vi "Run.vi"(8 "error in (no error)":errorcluster, 11 "Generic Plugin in":refnum<class "Generic Plugin.lvclass">) -> (0 "error out":errorcluster, 3 "Generic Plugin out":refnum<class "Generic Plugin.lvclass">)   [LabVIEW 2011, in "Generic Plugin.lvclass"]
uses:
  Generic Plugin.lvclass
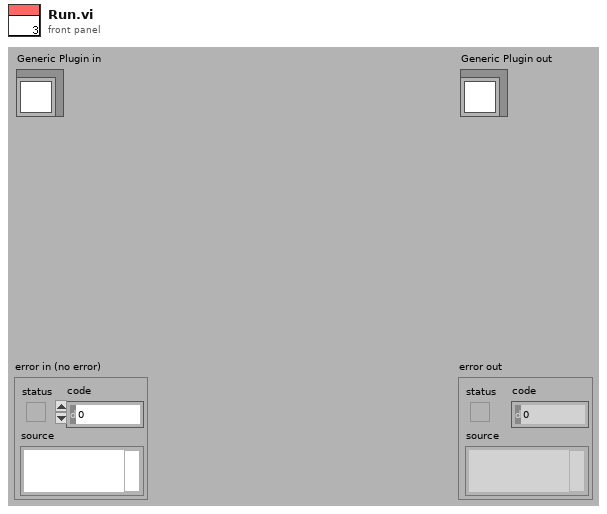
[diagram p1: front panel]
types:
  T1 = enum32{"Bad", "Idle", "Run top level", "Running"}
  T2 = cluster{"queue out":refnum<queue>, "Generic Plugin out":refnum<class "Generic Plugin.lvclass">}
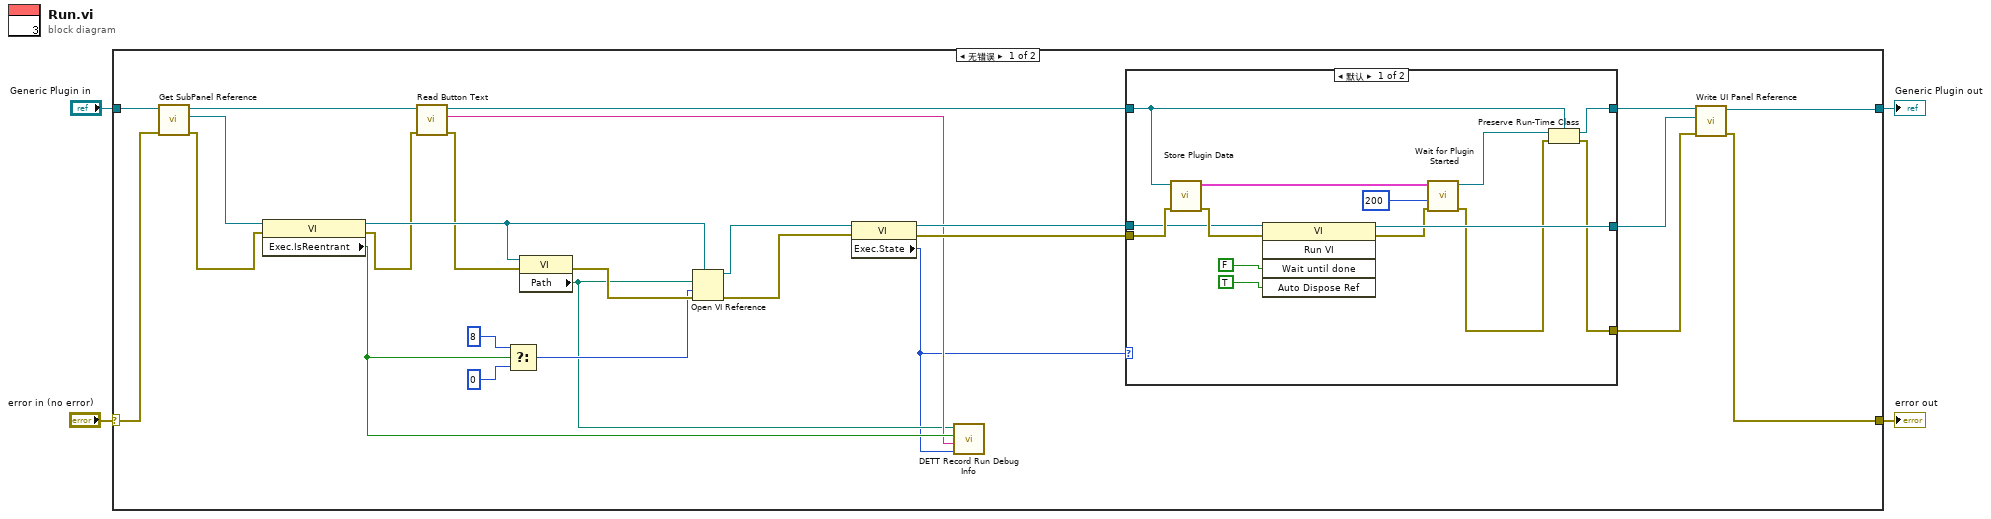
[diagram p0: block diagram]
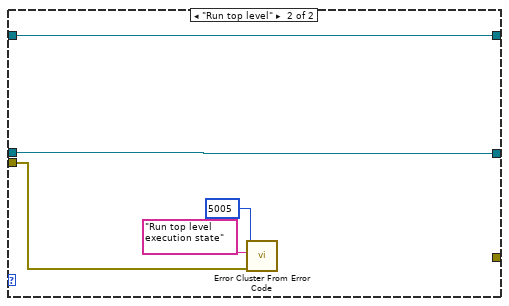
[diagram p2: hidden frame]
diagram:
  n1 = case shown="无错误" "error in (no error)" {
    selector: "error in (no error)" -> [w27 w51]
    tunnel: [w15 w51] -> w1
    tunnel: [w18 w50] -> w2
    tunnel: "Generic Plugin in" -> [w28 w50]
    frame No Error {
      n2 = call-dynamic "Get SubPanel Reference.vi"("error in (no error)"=w27, "Generic Plugin in"=w28) -> ("error out"=w8:errorcluster, "VI Ref"=w24:refnum<vi>, "Generic Plugin out"=w10:refnum<class "Generic Plugin.lvclass">)  [unwired: 7 in]
      n3 = property class="VI"(reference=w24, error in=w8) -> (reference out=w23:refnum<vi>, error out=w7:errorcluster, "Exec.IsReentrant"=w13:bool)
      n4 = call-dynamic "Read Button Text.vi"("error in (no error)"=w7, "Generic Plugin in"=w10) -> ("error out"=w6:errorcluster, "Button Text"=w12:string, "Generic Plugin out"=w9:refnum<class "Generic Plugin.lvclass">)  [unwired: 7 in]
      n5 = Select(t=8 ("options"), s=w13, f=0 ("options")) -> (s? t:f=w14:i32)
      n6 = property class="VI"(reference=w23, error in=w6) -> (error out=w26:errorcluster, "Path"=w11:path)  [unwired: 1 out]
      n7 = Open VI Reference(type specifier VI Refnum (for type only)=w23, vi path=w11, options=w14, error in (no error)=w26) -> (vi reference=w20:refnum<vi>, error out=w25:errorcluster)  [unwired: 2 in]
      n8 = property class="VI"(reference=w20, error in=w25) -> (reference out=w30:refnum<vi>, error out=w29:errorcluster, "Exec.State"=w5:T1)
      n9 = call "DETT Record Run Debug Info.vi"("Exec.State"=w5, "Button Text"=w12, "Exec.IsReentrant"=w13, "Path"=w11) -> ()
      n10 = case shown="默认" w5 {
        tunnel: w30 -> [w37 w49]
        tunnel: w29 -> [w41 w45]
        tunnel: [w31 _] -> w16
        tunnel: [w42 w49] -> w17
        tunnel: w9 -> [w33 w48]
        tunnel: [w34 w48] -> w19
        frame Default {
          n11 = call "Store Plugin Data.vi"("error in (no error)"=w41, "Generic Plugin out"=w33) -> ("error out"=w40:errorcluster, "output cluster"=w36:T2)  [unwired: 8 in]
          n12 = invoke class="VI" method="Run VI"(reference=w37, error in=w40, "Wait until done"=FALSE ("Wait Until Done"), "Auto Dispose Ref"=TRUE ("Auto Dispose Reference")) -> (reference out=w42:refnum<vi>, error out=w39:errorcluster)  [unwired: 1 in, 3 out]
          n13 = call "Wait for Plugin Started.vi"("error in (no error)"=w39, "Timeout (ms)"=200, "pCOMM Ref 2"=w36) -> ("error out"=w32:errorcluster, "Generic Plugin out"=w35:refnum<class "Generic Plugin.lvclass">)  [unwired: 7 in]
          n14 = Preserve Run-Time Class(object in=w35, error in=w32, 2:w33) -> (object out=w34:refnum<class "Generic Plugin.lvclass">, error out=w31:errorcluster)
        }
        frame "Run top level" {
          n15 = call <vilib>:"Error Cluster From Error Code.vi"("error in (no error)"=w45, "error message (\"\")"="Run top level execution state" ("error message (\"\")"), "error code (0)"=5005) -> ()  [unwired: 6 in, 1 out]
        }
      }
      n16 = call "Write UI Panel Reference.vi"("error in (no error)"=w16, "UI Panel Reference"=w17, "Generic Plugin in"=w19) -> ("error out"=w15:errorcluster, "Generic Plugin out"=w18:refnum<class "Generic Plugin.lvclass">)  [unwired: 7 in]
    }
    frame Error {
    }
  }
  "error out" <- w1
  "Generic Plugin out" <- w2
